vi "Server(XML).vi"() -> ()   [LabVIEW 2013, in "OPC UA Demo.lvlib"]
doc: "Demonstrates the use of the <B>OPC UA Server</B> VIs to programmatically create an OPC UA server."
uses:
  OPC UA Demo.lvlib
  <vilib>/OPCUA/server/Write Int32.vi
  <vilib>/OPCUA/server/Read Int32.vi
  <vilib>/OPCUA/NI OPC UA Server.lvlib
  OPCUA XML/OPCUA XML.lvlib
panel:
  out "Device.Node.Set Point":i32
  out "Device.Node":i32
  out "server endpoint URL":string
  out "error out":errorcluster
  in  "stop":bool
  # "Overview: Demonstrates the use of the OPC UA Server VIs to programmatically create an OPC UA server.\nRequirements: \n1. LabVIEW Datalogging and Supervisory Control Module or LabVIEW Real-Time Module\n2. (Real-Time Module) RT target\nInstructions:\nRun the VI."
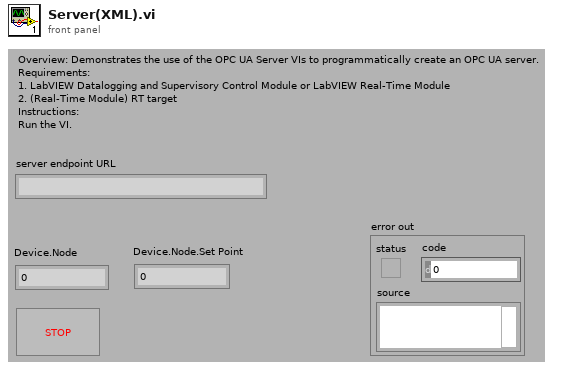
[diagram p1: front panel]
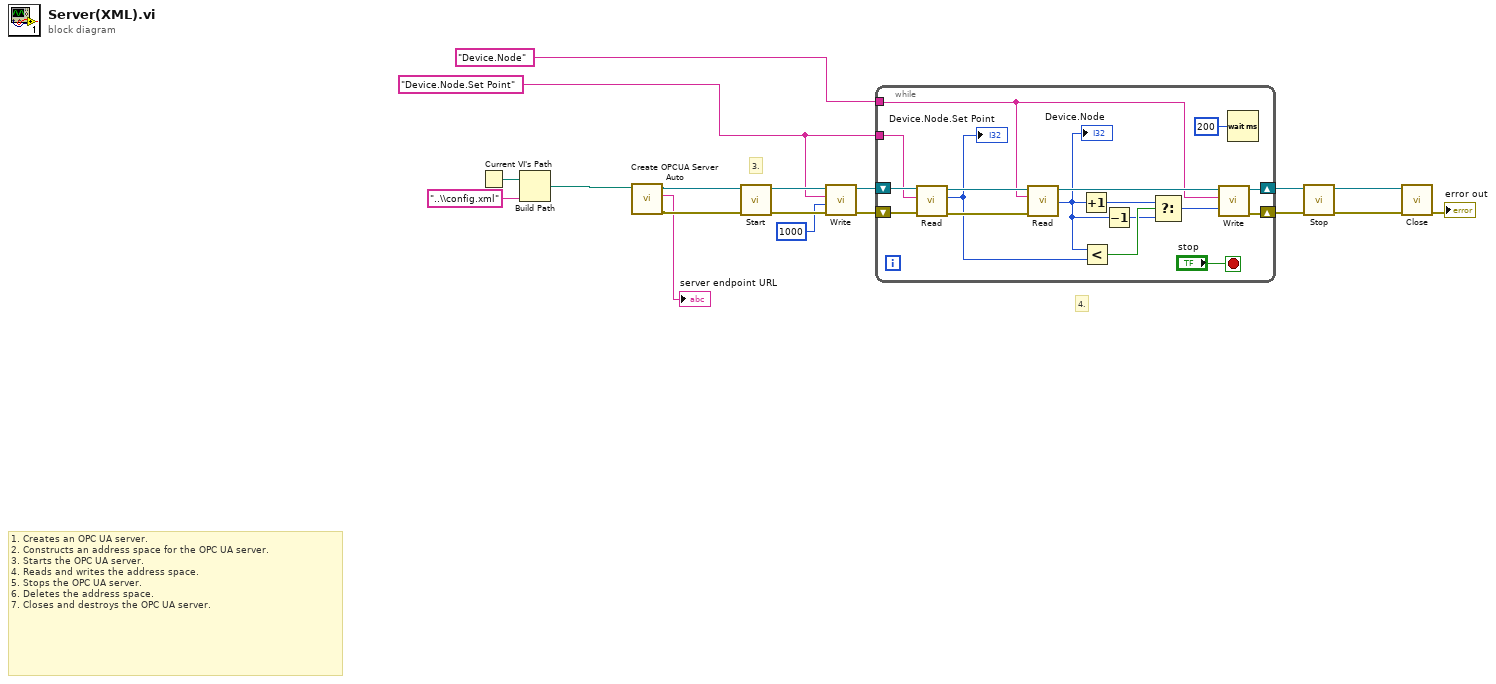
[diagram p0: block diagram]
diagram:
  w10 = "Device.Node.Set Point" ("property path")
  # "1. Creates an OPC UA server.\n2. Constructs an address space for the OPC UA server.\n3. Starts the OPC UA server.\n4. Reads and writes the address space.\n5. Stops the OPC UA server.\n6. Deletes the address space.\n7. Closes and destroys the OPC UA server."
  # "4."
  # "3."
  n1 = Current VI's Path() -> (path=w12:path)
  n2 = Build Path(base path=w12, name or relative path="..\\config.xml") -> (appended path=w6:path)
  n3 = call "Create OPCUA Server Auto.vi"("XML config File Path"=w6) -> ("Error Out"=w7:errorcluster, "server endpoint URL"=→"server endpoint URL":string, "OPC UA server refnum out"=w8:refnum<k21>)  [unwired: 6 in, 2 out]
  n4 = call <vilib>:"Start.vi"("error in (no error)"=w7, "OPC UA server refnum in"=w8) -> ("error out"=w15:errorcluster, "OPC UA server refnum out"=w18:refnum<k21>)  [unwired: 8 in]
  n5 = call-poly <vilib>:"Write.vi"("error in (no error)"=w15, "value"=1000, "node path"=w10, "OPC UA server refnum in"=w18) -> ("error out"=w14:errorcluster, "OPC UA server refnum out"=w16:refnum<k21>)  [unwired: 6 in]
  n6 = while {
    tunnel: "Device.Node" ("item path") -> [w25]
    shift-right: [w31] -> w4
    shift-left: w16 -> [w30]
    shift-right: [w29] -> w1
    shift-left: w14 -> [w33]
    tunnel: w10 -> [w28]
    stop <- "stop" stop-if-true
    n7 = call-poly <vilib>:"Read.vi"("error in (no error)"=w33, "node path"=w28, "OPC UA server refnum in"=w30) -> ("error out"=w26:errorcluster, "value"=w24:i32, "OPC UA server refnum out"=w34:refnum<k21>)  [unwired: 4 in, 2 out]
    "Device.Node.Set Point" <- w24
    n8 = call-poly <vilib>:"Read.vi"("error in (no error)"=w26, "node path"=w25, "OPC UA server refnum in"=w34) -> ("value"=w20:i32, "OPC UA server refnum out"=w27:refnum<k21>)  [unwired: 4 in, 3 out]
    "Device.Node" <- w20
    n9 = Increment(x=w20) -> (x+1=w22:i32)
    n10 = Less?(x=w20, y=w24) -> (x < y?=w23:bool)
    n11 = Decrement(x=w20) -> (x-1=w21:i32)
    n12 = Select(t=w22, s=w23, f=w21) -> (s? t:f=w19:i32)
    n13 = call-poly <vilib>:"Write.vi"("value"=w19, "node path"=w25, "OPC UA server refnum in"=w27) -> ("error out"=w29:errorcluster, "OPC UA server refnum out"=w31:refnum<k21>)  [unwired: 7 in]
    n14 = Wait (ms)(milliseconds to wait=u32 200) -> ()  [unwired: 1 out]
  }
  n15 = call <vilib>:"Stop.vi"("error in (no error)"=w1, "OPC UA server refnum in"=w4) -> ("error out"=w2:errorcluster, "OPC UA server refnum out"=w3:refnum<k21>)  [unwired: 8 in]
  n16 = call <vilib>:"Close.vi"("error in (no error)"=w2, "OPC UA server refnum in"=w3) -> ("error out"=→"error out":errorcluster)  [unwired: 9 in]
